vi "move.vi"(8 "error in":errorcluster, 9 "Relative? (T)":bool=TRUE, 10 "Destination (steps)":i16, 11 "Newport Model 8742 in":refnum<class "New Focus Model 8742.lvclass">) -> (0 "error out":errorcluster, 3 "Newport Model 8742 out":refnum<class "New Focus Model 8742.lvclass">)   [LabVIEW 2020, in "New Focus Model 8742.lvclass"]
uses:
  New Focus Model 8742.lvclass
  New Focus Model 8742.lvclass/New Focus Model 8742.ctl
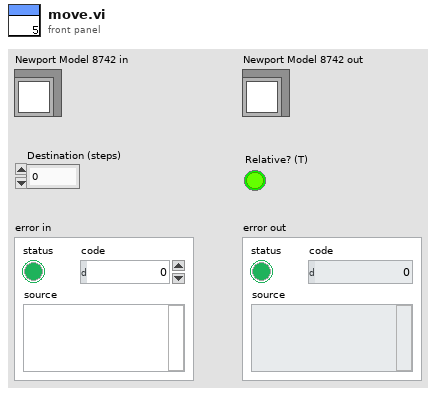
[diagram p1: front panel]
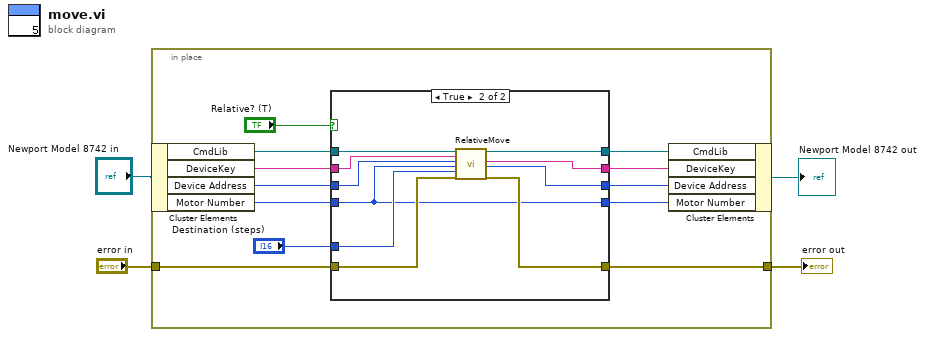
[diagram p0: block diagram]
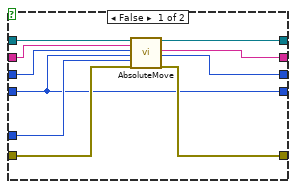
[diagram p2: hidden frame]
diagram:
  n1 = in-place {
    in-place-border: "error in" -> [w11]
    in-place-border: [w6] -> w1
    n2 = in-place-cluster #1("Newport Model 8742 in") -> ("CmdLib"=w15:refnum<k24>, "DeviceKey"=w14:string, "Device Address"=w13:i32, "Motor Number"=w12:i32)
    n3 = case shown="True" "Relative? (T)" {
      tunnel: w15 -> [w26 w35]
      tunnel: w14 -> [w25 w34]
      tunnel: w13 -> [w24 w33]
      tunnel: w12 -> [w17 w27]
      tunnel: w11 -> [w22 w36]
      tunnel: "Destination (steps)" -> [w23 w32]
      tunnel: [w21 w31] -> w9
      tunnel: [w20 w30] -> w8
      tunnel: [w19 w29] -> w7
      tunnel: [w18 w28] -> w6
      tunnel: [w17 w27] -> w5
      frame False {
        n4 = call <instrlib>:"AbsoluteMove.vi"("CmdLib In"=w26, "DeviceKey In"=w25, "Device Address In"=w24, "Motor"=w17, "Target Pos"=w23, "error in (no error)"=w22) -> ("CmdLib Out"=w21:refnum<k24>, "DeviceKey Out"=w20:string, "Device Address Out"=w19:i32, "error out"=w18:errorcluster)  [unwired: 10 in]
      }
      frame True {
        n5 = call <instrlib>:"RelativeMove.vi"("CmdLib In"=w35, "DeviceKey In"=w34, "Device Address In"=w33, "Motor"=w27, "Relative Steps"=w32, "error in (no error)"=w36) -> ("CmdLib Out"=w31:refnum<k24>, "DeviceKey Out"=w30:string, "Device Address Out"=w29:i32, "error out"=w28:errorcluster)  [unwired: 10 in]
      }
    }
    n6 = in-place-cluster #1("CmdLib"=w9, "DeviceKey"=w8, "Device Address"=w7, "Motor Number"=w5) -> (→"Newport Model 8742 out":refnum<class "New Focus Model 8742.lvclass">)
  }
  "error out" <- w1
